vi "RSZVB Get Loss Reference Frequency.vi"(8 "error in (no error)":errorcluster {"code" format="%.0x"}, 9 "Port (1)":i32=1, 10 "Channel (1)":i32=1, 11 "VISA session":refnum<visa-resource-name>) -> (0 "error out":errorcluster {"code" format="%.0x"}, 1 "Loss Reference Frequency":dbl format="%^.3e", 3 "dup VISA session":refnum<visa-resource-name>)   [LabVIEW 2011]
doc: "This VI returns the reference frequency for the frequency-dependent part of the offset loss ([SENSe<Ch>:]CORRection:LOSS<port_no>:OFFSet).\n\nRemote-control command(s):\n[SENSe<Ch>:]CORRection:LOSS<port_no>:FREQuency?"
uses:
  _utility/RSZVB Global Data.vi
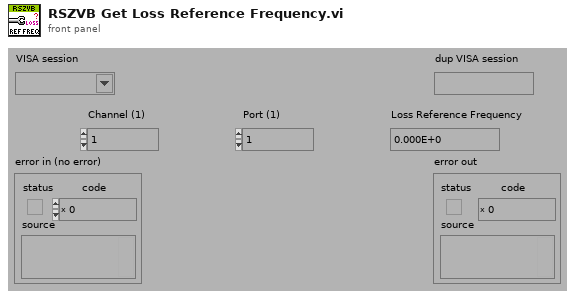
[diagram p1: front panel]
types:
  T1 = cluster{"Error Checking (T: On)":bool, "Installed Options":string[], "Data Valid?":bool, "Ports":i32, "Model":string[], "Option Checking (T: On)":bool}[]
  T2 = cluster{"Error Checking (T: On)":bool, "Installed Options":string[], "Data Valid?":bool, "Ports":i32, "Model":string[], "Option Checking (T: On)":bool}
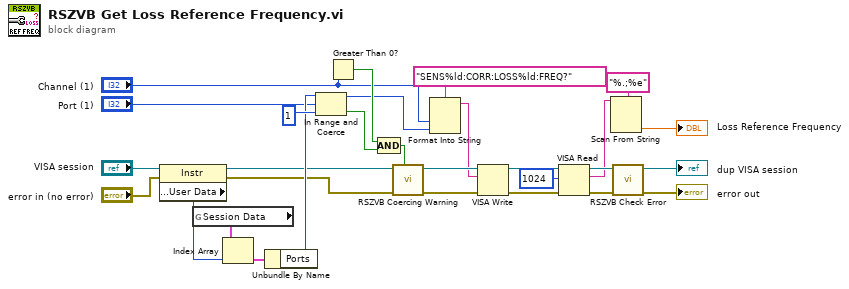
[diagram p0: block diagram]
diagram:
  n1 = property class="Instr"(reference="VISA session", error in="error in (no error)") -> (reference out=w17:refnum<visa-resource-name>, error out=w18:errorcluster, "General Settings:User Data"=w21:u32)
  n2 = global read "RSZVB Global Data.vi" "Session Data"() -> (w22:T1)
  n3 = Index Array(array=w22, index=w21) -> (element=w23:T2)
  n4 = Unbundle By Name(w23) -> ("Ports"=w19:i32)
  n5 = In Range and Coerce(upper limit=w19, x="Port (1)", lower limit=1) -> (coerced(x)=w16:i32, In Range?=w15:bool)
  n6 = Greater Than 0?(x="Channel (1)") -> (x > 0?=w24:bool)
  n7 = Compound Arithmetic op=AND(w24, w15) -> (w26:bool)
  n8 = call "RSZVB Coercing Warning.vi"("In Range?"=w26, "error in (no error)"=w18, "VISA session"=w17) -> ("error out"=w27:errorcluster, "dup VISA session"=w28:refnum<visa-resource-name>)  [unwired: 7 in]
  n9 = Format Into String(format string="SENS%ld:CORR:LOSS%ld:FREQ?", "Channel (1)", w16) -> (resulting string=w25:string)  [unwired: 2 in, 1 out]
  n10 = VISA Write(VISA resource name=w28, write buffer=w25, error in (no error)=w27) -> (VISA resource name out=w9:refnum<visa-resource-name>, error out=w8:errorcluster)  [unwired: 1 out]
  n11 = VISA Read(VISA resource name=w9, byte count=u32 1024 ("byte count (0)"), error in (no error)=w8) -> (VISA resource name out=w14:refnum<visa-resource-name>, read buffer=w11:string, error out=w13:errorcluster)  [unwired: 1 out]
  n12 = Scan From String(format string="%.;%e", input string=w11) -> (output 1=→"Loss Reference Frequency":dbl)  [unwired: 3 in, 3 out]
  n13 = call "RSZVB Check Error.vi"("error in (no error)"=w13, "VISA session"=w14) -> ("error out"=→"error out":errorcluster, "dup VISA session"=→"dup VISA session":refnum<visa-resource-name>)  [unwired: 8 in]
